vi "FT_Write_String_Data.vi"(0 "Handle":u32, 1 "Buffer":string) -> (2 "FT_Status":u32, 3 "Bytes Written":u32, 4 "Handle":u32, 5 "Buffer out":string)   [LabVIEW 2011]
uses:
  FTD2XX.dll
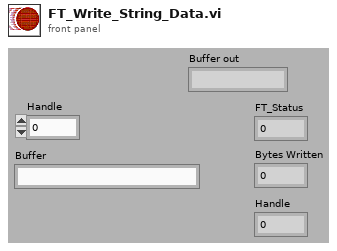
[diagram p1: front panel]
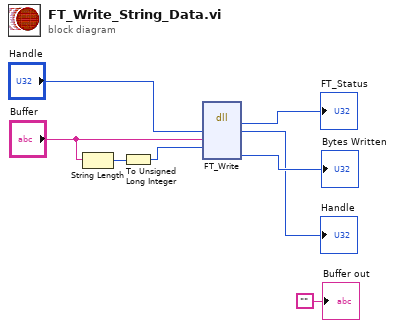
[diagram p0: block diagram]
diagram:
  n1 = String Length(string="Buffer") -> (length=w4:i32)
  n2 = To Unsigned Long Integer(number=w4) -> (unsigned 32bit integer=w3:u32)
  n3 = dll-call lib="C:/Work/Labview/#Avesta/D2XX_Functions_7.0/FTD2XX.dll" fn="FT_Write"("Handle"="Handle", "Buffer"="Buffer", "BytesToWrite"=w3) -> ("FT_Status"=→"FT_Status":u32, "Handle"=→"Handle":u32, "BytesWritten"=→"Bytes Written":u32)  [unwired: 5 in, 3 out]
  "Buffer out" <- ""
